vi "SubPanel_PowerConfiguration_Rev11_v4.vi"(3 "error in":errorcluster, 4 "VISAPowerInfoInputArray":T2[](array[typedef]), 5 "DCPowerInformationClusterArray_Input":T1[](array[typedef])) -> (0 "error out":errorcluster, 1 "VISAPowerInfoOutputArray":T2[](array[typedef]), 2 "DCPowerInformationClusterArray_Output":T1[](array[typedef]))   [LabVIEW 2019]
uses:
  Controls/PlotColorArray.ctl
  Controls/VISA_power_Control.ctl
  Controls/DCPowerBlock_byInstrument_Control.ctl
panel:
  out "DCPowerInformationClusterArray":T1[](array[typedef])
  out "VISAPowerInformationClusterArray":T2[](array[typedef])
  out "Current Measurement (A)":dbl[][](array[numeric])
  out "Voltage Measurement (V)":dbl[][](array[numeric])
  out "Voltage Waveform Array":waveform(dbl)[](graph)
  out "Current Waveform Array":waveform(dbl)[](graph)
  out "Supplies Updated?":bool
  in  "Update Changes":bool
  out "VISAPowerInformationClusterOutput":T3(array[cluster])
  in  "Exit SubVI":bool
  in  "Instrument Cards (Must Reconfigure if you add new cards or change the names in NI Max)":T4(tab)
  in  "VISA resource name":refnum<visa-resource-name>
  in  "Apply Power Settings":bool
  out "POWER STATUS":bool
  in  "POWER ON":bool
  in  "Voltage Channel 1":dbl
  in  "Voltage Channel 2":dbl
  in  "Voltage Channel 3":dbl
  in  "Current Limit Channel 1":dbl
  in  "Current Limit Channel 2":dbl
  in  "Current Limit Channel 3":dbl
  out "Parameter Configuration Echo":string[][](array[string])
  out "Configuration Echo":string
  in  "Which Channels to Parallelize":u16(ring) items=["I1+I2", "ALL", "I2+I3"]
  in  "Combination Scheme":u16(ring) items=["OFF", "SERIES", "PARALLEL"]
  in  "Current Reset Value 23":dbl
  in  "Current Reset Value 22":dbl
  in  "Current Reset Value 21":dbl
  in  "Current Reset Value 20":dbl
  in  "Current Reset Value 19":dbl
  in  "Current Reset Value 18":dbl
  in  "Current Reset Value 17":dbl
  in  "Current Reset Value 16":dbl
  in  "Current Reset Value 15":dbl
  in  "Current Reset Value 14":dbl
  in  "Current Reset Value 13":dbl
  in  "Current Reset Value 12":dbl
  in  "Current Reset Value 11":dbl
  in  "Current Reset Value 10":dbl
  in  "Current Reset Value 9":dbl
  in  "Current Reset Value 8":dbl
  in  "Current Reset Value 7":dbl
  in  "Current Reset Value 6":dbl
  in  "Current Reset Value 5":dbl
  in  "Current Reset Value 4":dbl
  in  "Current Reset Value 3":dbl
  in  "Current Reset Value 2":dbl
  in  "Current Reset Value 1":dbl
  in  "voltage level channel 26":dbl caption="voltage level channel 0" format="%.6p"
  in  "voltage level channel 1":dbl format="%.6p"
  in  "voltage level channel 2":dbl format="%.6p"
  in  "voltage level channel 3":dbl format="%.6p"
  in  "voltage level channel 4":dbl format="%.6p"
  in  "voltage level channel 5":dbl format="%.6p"
  in  "voltage level channel 6":dbl format="%.6p"
  in  "voltage level channel 7":dbl format="%.6p"
  in  "voltage level channel 8":dbl format="%.6p"
  in  "voltage level channel 9":dbl format="%.6p"
  in  "voltage level channel 10":dbl format="%.6p"
  in  "voltage level channel 11":dbl format="%.6p"
  in  "voltage level channel 12":dbl format="%.6p"
  in  "voltage level channel 13":dbl format="%.6p"
  in  "voltage level channel 14":dbl format="%.6p"
  in  "voltage level channel 15":dbl format="%.6p"
  in  "voltage level channel 16":dbl format="%.6p"
  in  "voltage level channel 17":dbl format="%.6p"
  in  "voltage level channel 18":dbl format="%.6p"
  in  "voltage level channel 19":dbl format="%.6p"
  in  "voltage level channel 20":dbl format="%.6p"
  in  "voltage level channel 21":dbl format="%.6p"
  in  "voltage level channel 22":dbl format="%.6p"
  in  "voltage level channel 23":dbl format="%.6p"
  in  "Activate Channel 0":bool
  in  "Activate Channel 1":bool
  in  "Activate Channel 2":bool
  in  "Activate Channel 3":bool
  in  "Activate Channel 4":bool
  in  "Activate Channel 5":bool
  in  "Activate Channel 6":bool
  in  "Activate Channel 7":bool
  in  "Activate Channel 8":bool
  in  "Activate Channel 9":bool
  in  "Active Channel 10":bool
  in  "Activate Channel 11":bool
  in  "Activate Channel 12":bool
  in  "Activate Channel 13":bool
  in  "Activate Channel 14":bool
  in  "Activate Channel 15":bool
  in  "Activate Channel 16":bool
  in  "Activate Channel 17":bool
  in  "Activate Channel 18":bool
  in  "Activate Channel 19":bool
  in  "Activatate Channel 20":bool
  in  "Activate Channel 21":bool
  in  "Activate Channel 22":bool
  in  "Activate Channel 23":bool
  in  "Channel Name 0":string="NULL0"
  in  "Channel Name 1":string="NULL1"
  in  "Channel Name 2":string="NULL2"
  in  "Channel Name 3":string="NULL3"
  in  "Channel Name 4":string="NULL4"
  in  "Channel Name 5":string="NULL5"
  in  "Channel Name 6":string="NULL6"
  in  "Channel Name 7":string="NULL7"
  in  "Channel Name 8":string="NULL8"
  in  "Channel Name 9":string="NULL9"
  in  "Channel Name 10":string="NULL10"
  in  "Channel Name 11":string="NULL11"
  in  "Channel Name 12":string="NULL12"
  in  "Channel Name 13":string="NULL13"
  in  "Channel Name 14":string="NULL14"
  in  "Channel Name 15":string="NULL15"
  in  "Channel Name 16":string="NULL16"
  in  "Channel Name 17":string="NULL17"
  in  "Channel Name 18":string="NULL18"
  in  "Channel Name 19":string="NULL19"
  in  "Channel Name 20":string="NULL20"
  in  "Channel Name 21":string="NULL21"
  in  "Channel Name 22":string="NULL22"
  in  "Channel Name 23":string="NULL23"
  in  "Apply Power Settings":bool
  in  "Aperture Time (s)":dbl=0.0001
  in  "Measure Record Length":i32=1000000
  in  "current limit (A) 2":dbl=0.05
  out "All Channel Numbers Array 2":string[](array[string])=["0", "1", "2", "3", "4", "5", "6", "7", "8", "9", "10", "11", "12", "13", "14", "15", "16", "17", "18", "19", "20", "21", "22", "23"]
  out "Active Channels Indicator 2":bool[](array[boolean])
  out "Voltage Array":dbl[](array[numeric])
  out "Active Channel Numbers Array 2":string[](array[string])
  out "Active Channel Voltage Array":dbl[](array[numeric])
  out "Active Channel Names Array":string[](array[string])
  in  "Current Reset Value 0":dbl
  in  "voltage level channel 0":dbl=1.0 format="%.6p"
  in  "Activate Channel 0":bool
  in  "Queue Power Settings":bool
  in  "Channel Name 0":string="NULL_0_slot16"
  out "Active Channel Voltage Array 3":dbl[](array[numeric])
  out "Active Channels Indicator 3":bool[](array[boolean])
  out "Voltage Array":dbl[](array[numeric])=[1.0]
  out "Active Channel Names Array":string[](array[string])
  out "Active Channel Numbers Array 3":string[](array[string])
  out "All Channel Numbers Array 3":string[](array[string])=["0"]
  in  "current limit (A) 3":dbl=3.0
  in  "Measure Record Length":i32=1000000
  in  "Aperture Time (s)":dbl=0.001
  in  "Current Reset Value 0":dbl
  in  "Queue Power Settings":bool
  in  "Aperture Time (s)":dbl=0.001
  in  "Measure Record Length":i32=1000000
  in  "current limit (A) 4":dbl=3.0
  in  "Activate Channel 0":bool
  in  "voltage level channel 0":dbl=2.0 format="%.6p"
  in  "Channel Name 0":string="NULL_0_slot_16"
  out "Active Channel Names Array":string[](array[string])
  out "Active Channel Voltage Array 4":dbl[](array[numeric])
  out "Active Channel Numbers Array 4":string[](array[string])
  out "Voltage Array":dbl[](array[numeric])=[2.0]
  out "Active Channels Indicator 4":bool[](array[boolean])
  out "All Channel Numbers Array 4":string[](array[string])=["0"]
  in  "Current Reset Value 0":dbl
  in  "Current Reset Value 0":dbl
  out "Active Channel Names Array":string[](array[string])
  out "Active Channel Voltage Array":dbl[](array[numeric])
  out "Active Channel Numbers Array":string[](array[string])
  out "Voltage Array":dbl[](array[numeric])=[3.0]
  out "All Channel Numbers Array":string[](array[string])=["0"]
  out "Active Channels Indicator":bool[](array[boolean])
  in  "voltage level channel 0":dbl=3.0 format="%.6p"
  in  "Activate Channel 0":bool
  in  "Channel Name 0":string="NULL_0_slot16"
  in  "Queue Power Settings":bool
  in  "Aperture Time (s)":dbl=0.001
  in  "Measure Record Length":i32=1000000
  in  "current limit (A)":dbl=3.0
  out "DCPowerInformationClusterOutput":T5(array[cluster])
  in  "ColorPalette":T6=[16711686, 65351, 8978420, 14474240, 16139007, 16752640, 8958719, 16758973, 16777215, 46792, 11992992, 12961221, 16763690, 12600063, 16711835, 2953983, 40796, 13111296, 13352613, 9221011, 12964076, 12819897, 65442, 16776704, 14540253, 16740729, 10658047, 10813344, 16753521, 13413843, 8691115, 10339240, 14401205, 16746704, 7467519, 16775978, 13872558, 11387603, 13354405, 10420227, 13107364, 4060, 35208, 11817216, 7566080, 40796, 7539456, 2837073, 6372186, 7499083, 10648702, 16757152]
  # "Background Information (Important)\nThis subvi has tabs that allow you to configure different power instruments. There are two options: VISA instruments or DC Power instruments. DC Power instruments are inside of the tester, visa instruments are external. If DCPower instruments are switched out, they will need to be reconfigured within the backend of this code (instructions pending). You are able to identify which channels you want to active, their individual voltage levels and the desired \"name\" of the channel (i.e. if you want channel 0 to be known at the \"ADMV1013_3p3V\" or \"GoodEnough\", you write it here). For the entire instrument, you can determine its capture rate (aperture time) or the current limit. I advise you do NOT alter the \"Measure Record Length\" as this is only if there are issues with the program. Shouldn't ever exceed this value. You apply the settings and they will be echoed back in each tab along with the array above. Multiple instruments can be configured and will show up as separate array elements\n\n\nInstructions (More Important):\n\nSelect instrument of interest (VISA KEITHLEY 2230G-30-6, PXIe-4163, and PXIe-4139 are the ones currently available). \n\n\nFOR DCPOWER INSTRUMENTS (PXI or PXIe)\n\nPress \"Active Channel #\" to select which channels you want to have power applied \n\nType in voltage level in \"Voltage level channel #\"\n\nType in desired channel name in \"Channel Name #\"\n\nType the measurement speed (suggest .0001) in aperture time\n\nType the current limit in \"current limit\"\n\nPress \"Apply Power Settings\" and review the echoed outputs within the tab and in the instrument array above the tabs.\n\nRepeat this process for other instruments\n\n\n\nFOR VISA INSTRUMENTS (NOT PXI or PXIe), note that it is case by case for instruments\n\nSelect resource name (you must know which one it is)\n\nPower on device if using it\n\nApply voltage settings \n\nApply current limits for each channel\n\nSelect which channels you will parallelize if at all\n\nSelect which combination scheme you will apply: OFF (individual channels), SERIES (Channel 1 and 2 in series), PARALLEL (I1 + I2, ALL, I2 + I3)\n\nFOR COMBINATIONS: for a combination scheme you choose, you only apply changes to the first channel of each. example: if you make the system series configuration, you only type you voltage information (i.e. 60V) into channel 1 and the current limit information into channel 1 but channel 3 is still independent of these\n\n\nPress \"Apply Powe Settings\" when complete\n\nReview the echoed values along with the instrument array above"
  # "All Voltage Level Channels are in Volts"
  # "Don't press enter when typing in strings. Just click out of it"
  # "Don't press enter when typing in strings. Just click out of it"
  # "Don't press enter when typing in strings. Just click out of it"
  # "Don't press enter when typing in strings. Just click out of it"
  # "Don't press enter when typing in strings. Just click out of it"
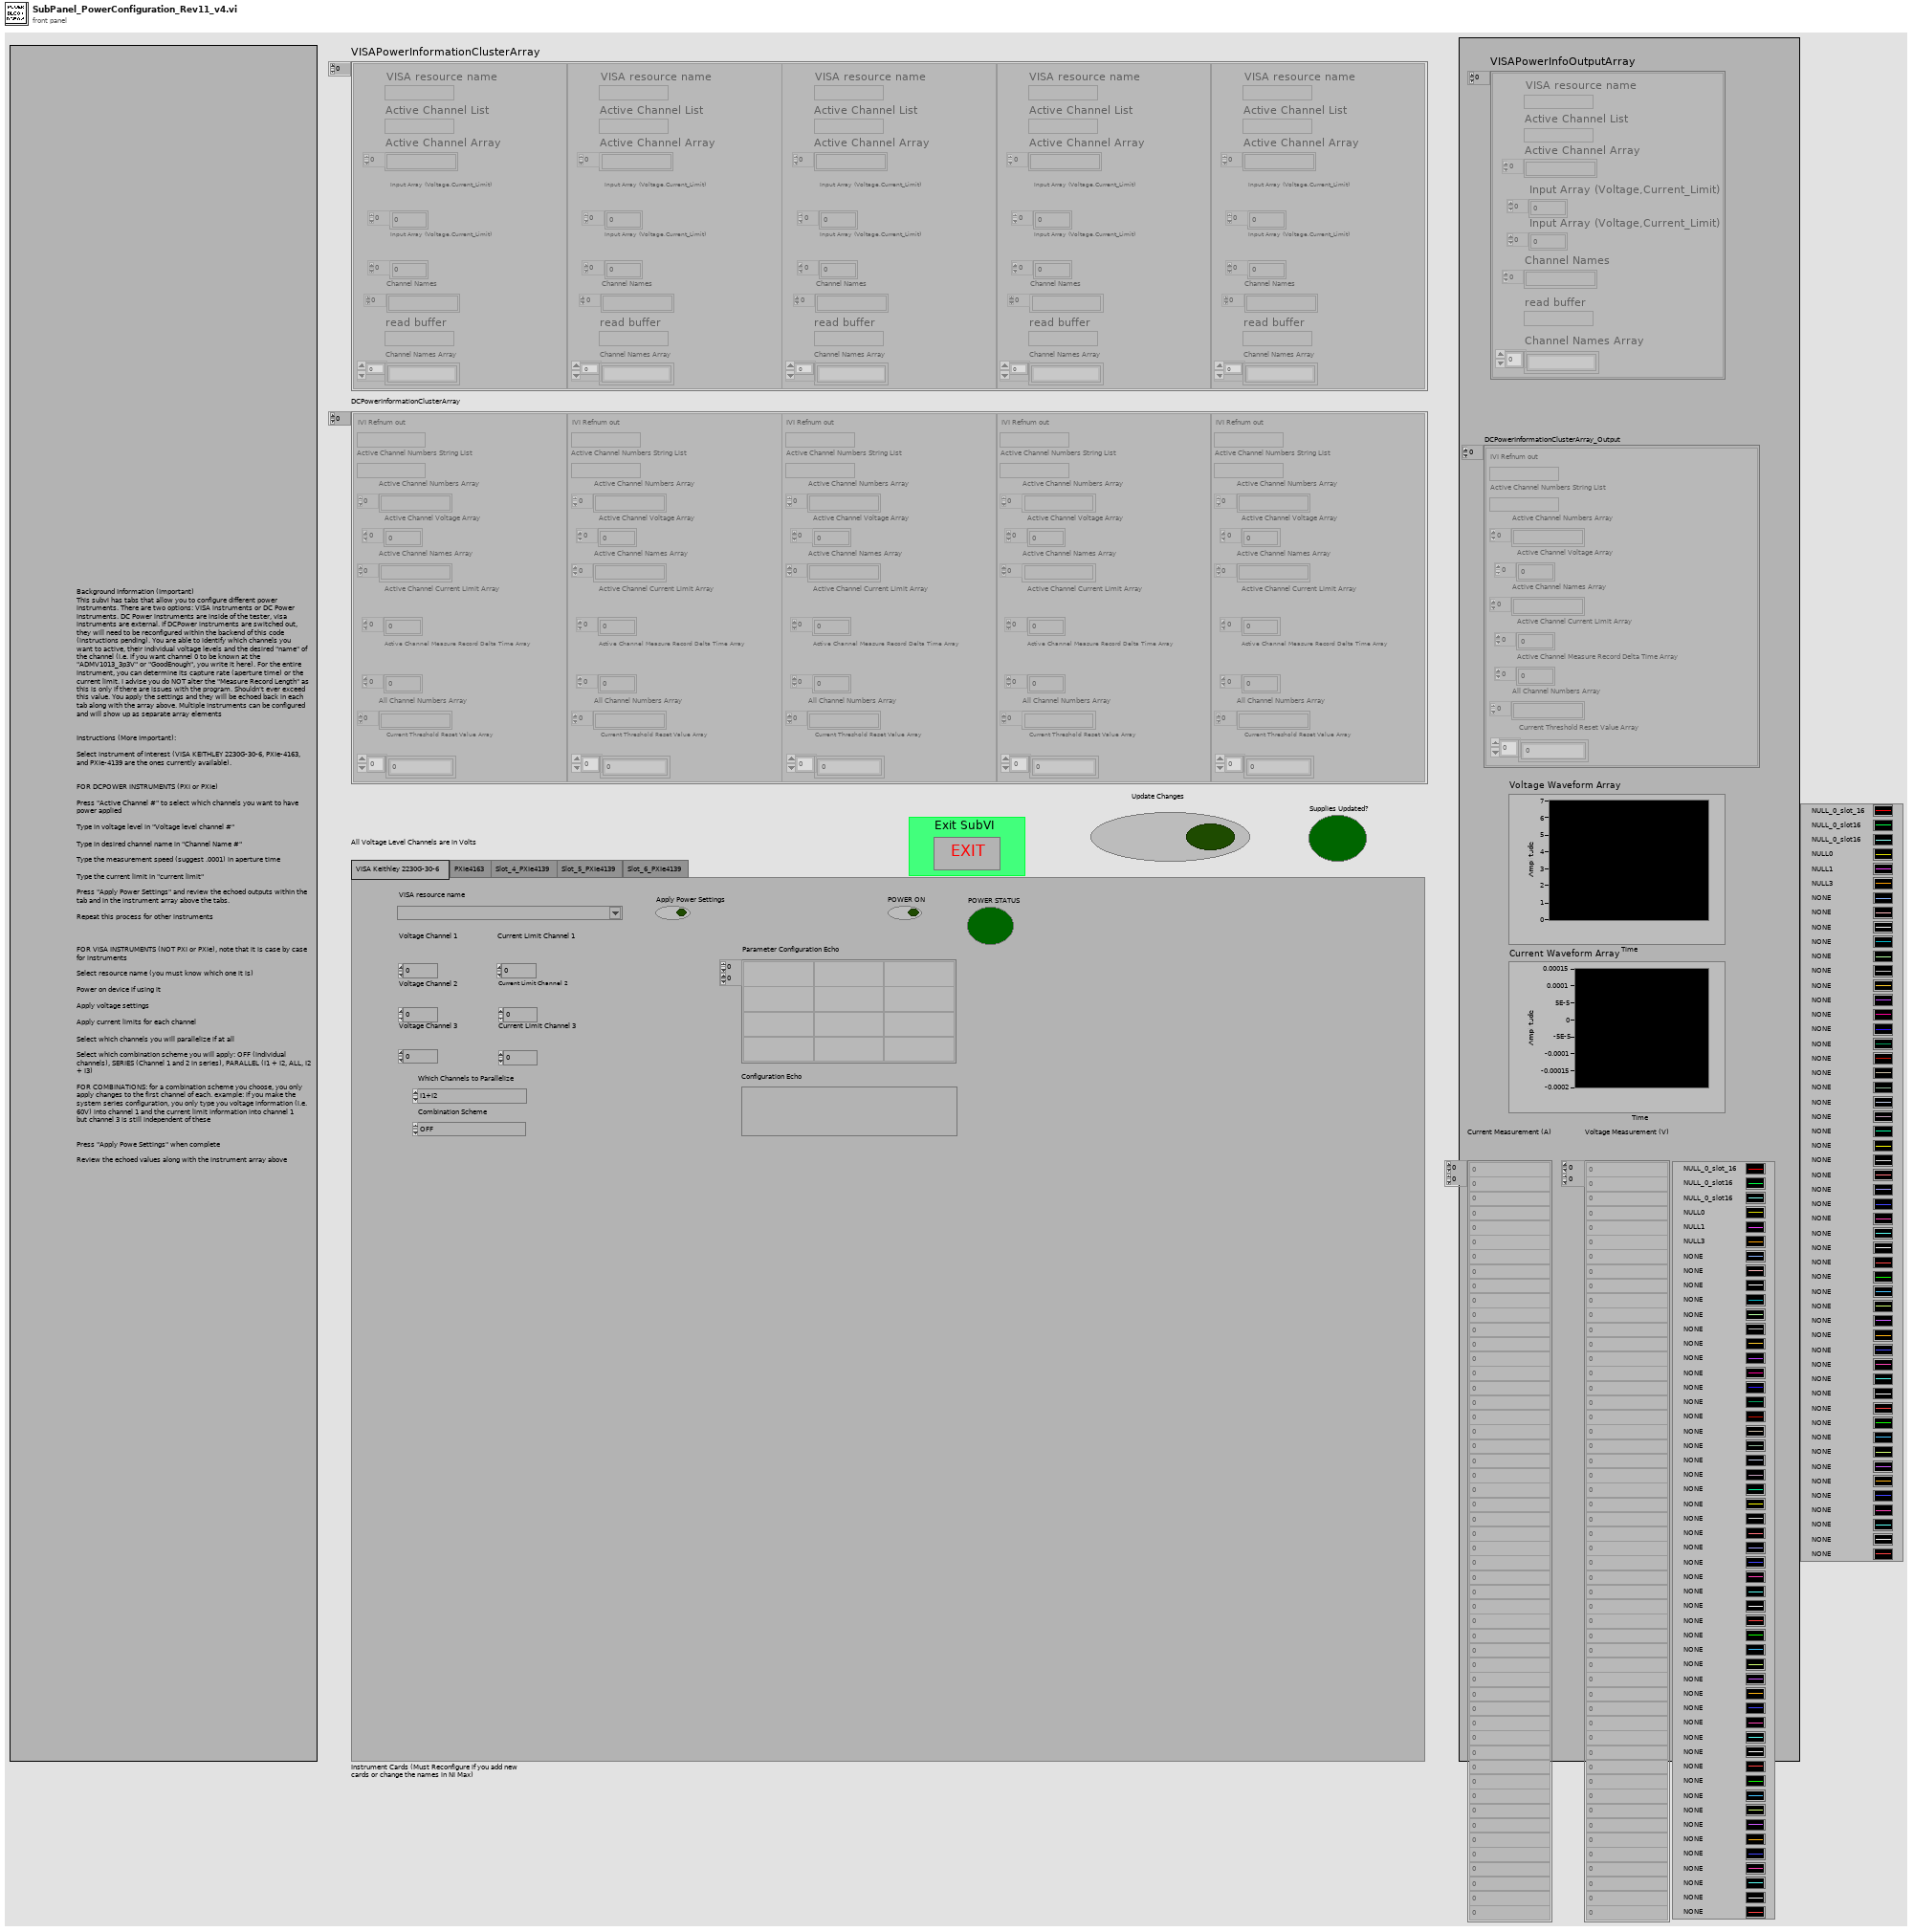
[diagram p1: front panel]
types:
  T1 = typedef "DCPowerBlock_byInstrument_Control.ctl" = cluster{"IVI Refnum out":refnum<k15>, "Active Channel Numbers String List":string, "Active Channel Numbers Array":string[], "Active Channel Voltage Array":dbl[], "Active Channel Names Array":string[], "Active Channel Current Limit Array":dbl[], "Active Channel Measure Record Delta Time Array":dbl[], "All Channel Numbers Array":string[], "Current Threshold Reset Value Array":dbl[]}
  T2 = typedef "VISA_power_Control.ctl" = cluster{"VISA resource name":refnum<visa-resource-name>, "Active Channel List":string, "Active Channel Array":string[], "Input Array (Voltage,Current_Limit)":dbl[], "Input Array (Voltage,Current_Limit)":dbl[], "Channel Names":string[], "read buffer":string, "Channel Names Array":string[]}
  T3 = cluster{"VISA resource name":refnum<visa-resource-name>, "String List":string, string[], "Input Array (Voltage,Current_Limit)":dbl[], "Input Array (Voltage,Current_Limit)":dbl[], "Channel Names":string[]}[]
  T4 = enum32{"VISA Keithley 2230G-30-6", "PXIe4163", "Slot_4_PXIe4139", "Slot_5_PXIe4139", "Slot_6_PXIe4139"}
  T5 = cluster{"instrument handle out":refnum<k15>, string, string[], dbl[], string[]}[]
  T6 = typedef "PlotColorArray.ctl" = u32[]
  T7 = cluster{"IVI Refnum out":refnum<k15>, "Active Channel Numbers String List":string, "Active Channel Numbers Array":string[], "Active Channel Voltage Array":dbl[], "Active Channel Names Array":string[], "Active Channel Current Limit Array":dbl[], "Active Channel Measure Record Delta Time Array":dbl[], "All Channel Numbers Array":string[]}[]
  T8 = cluster{"instrument handle out":refnum<k15>, string, string[], dbl[], string[], "Current Limit Output Array":dbl[], dbl[]}[]
  T9 = cluster{"IVI Refnum out":refnum<k15>, "Active Channel Numbers String List":string, "Active Channel Numbers Array":string[], "Active Channel Voltage Array":dbl[], "Active Channel Names Array":string[], "Active Channel Current Limit Array":dbl[], "Active Channel Measure Record Delta Time Array":dbl[], "All Channel Numbers Array":string[]}
  T10 = cluster{"VISA resource name":refnum<visa-resource-name>, "String List":string, string[], "Input Array (Voltage,Current_Limit)":dbl[], "Input Array (Voltage,Current_Limit)":dbl[], "Channel Names":string[], "read buffer":string}[]
  T11 = cluster{"IVI Refnum out":refnum<k15>, "Active Channel Numbers String List":string, "Active Channel Numbers Array":string[], "Active Channel Voltage Array":dbl[], "Active Channel Names Array":string[], "Active Channel Current Limit Array":dbl[], "Active Channel Measure Record Delta Time Array":dbl[], "aperture time string":string[], dbl[]}
  T12 = cluster{"IVI Refnum out":refnum<k15>, "Active Channel Numbers String List":string, "Active Channel Numbers Array":string[], "Active Channel Voltage Array":dbl[], "Active Channel Names Array":string[], "Active Channel Current Limit Array":dbl[], "Active Channel Measure Record Delta Time Array":dbl[], "All Channel Numbers Array":string[], dbl[]}
  T13 = cluster{"IVI Refnum out":refnum<k15>, string, "voltage level channel 23":dbl, "Channel Name 23":string, "Current Limit":dbl, "Measure Record dt":dbl, string, "Current Threshold Reset Value Array":dbl}[]
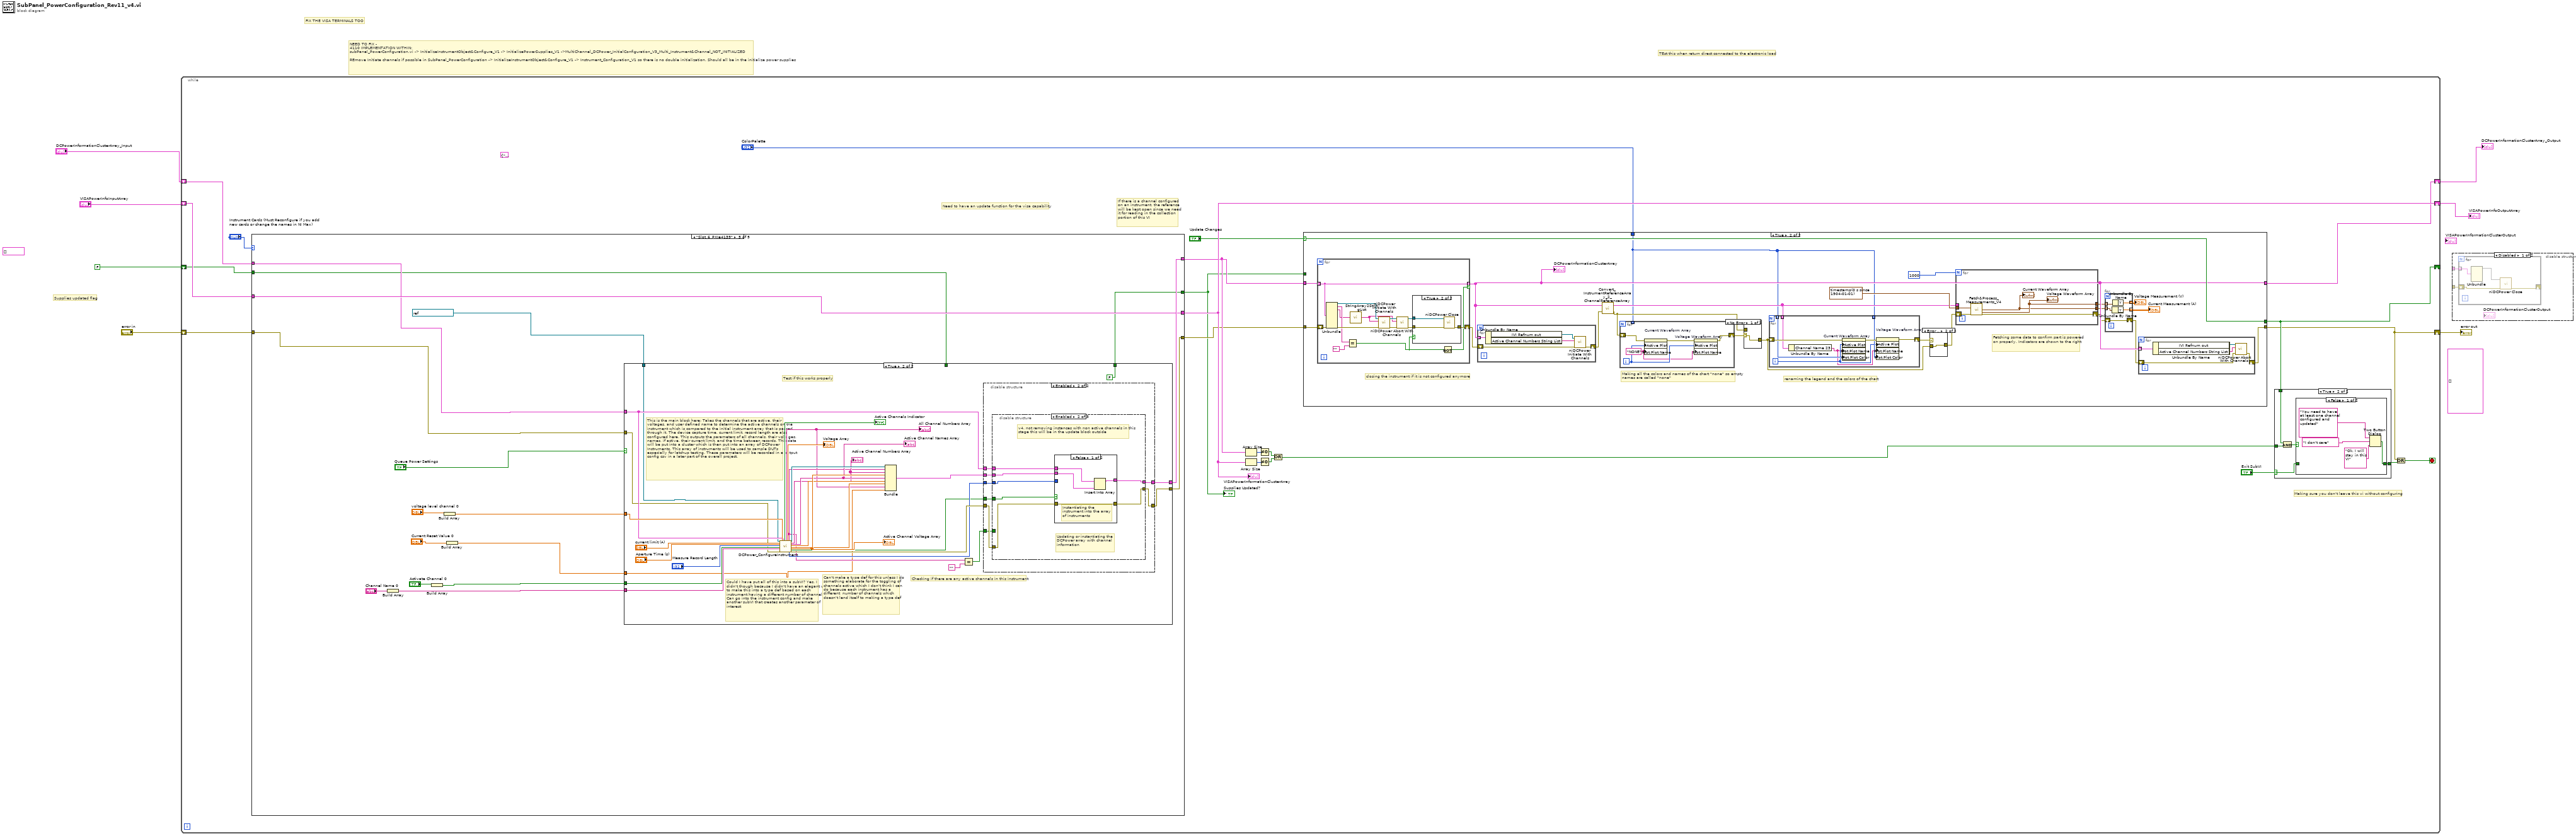
[diagram p0: block diagram]
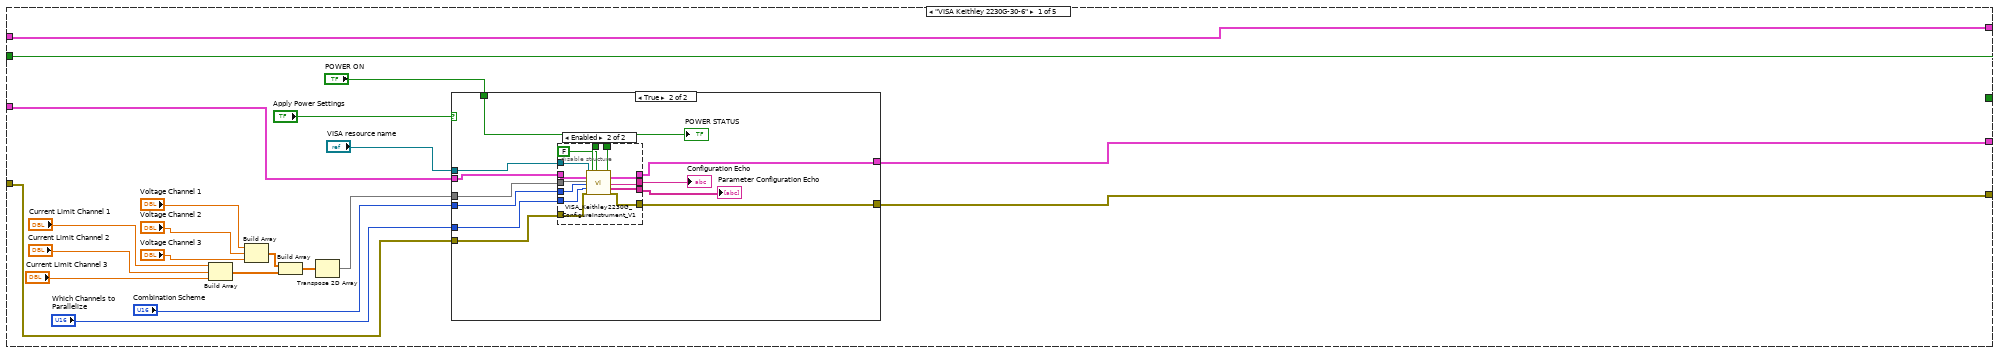
[diagram p9: hidden frame]
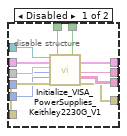
[diagram p11: hidden frame]
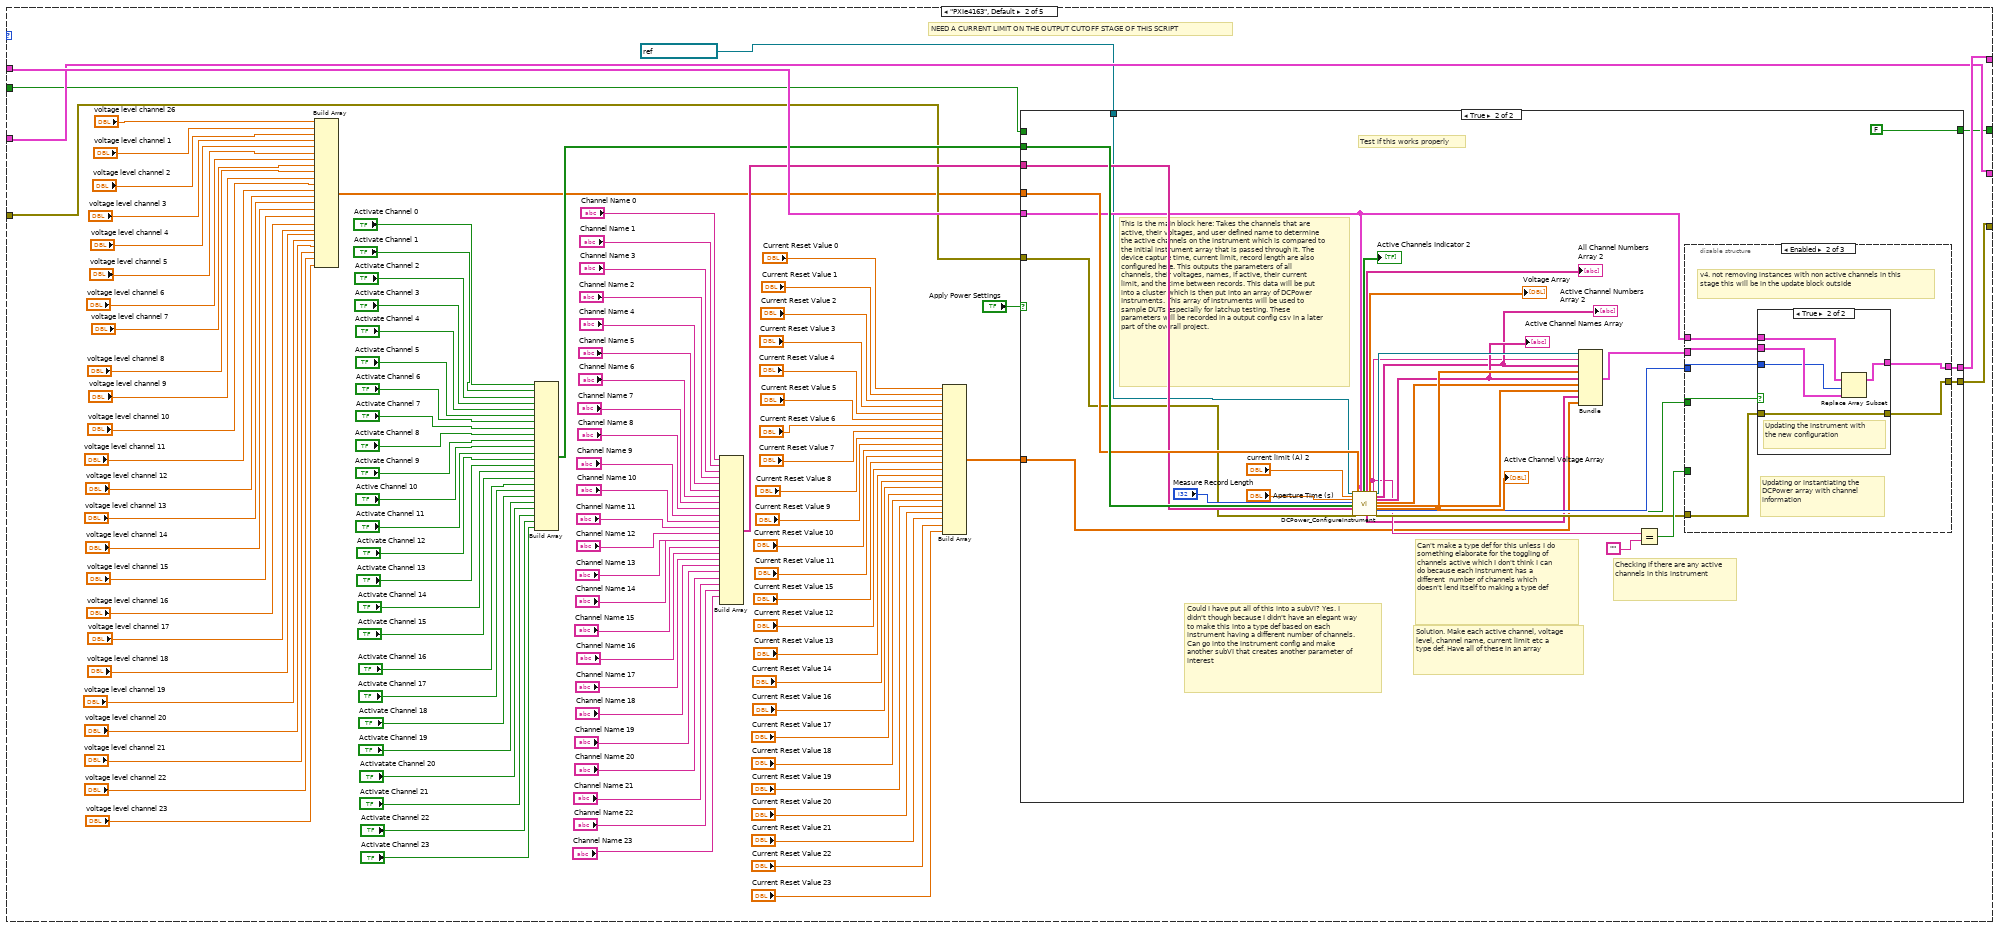
[diagram p12: hidden frame]
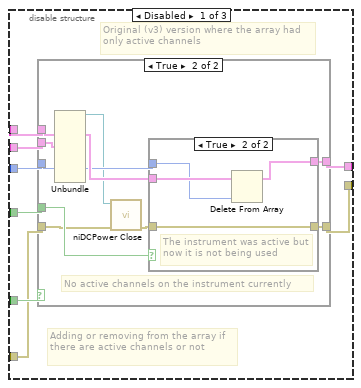
[diagram p14: hidden frame]
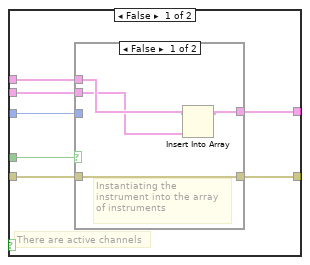
[diagram p15: hidden frame]
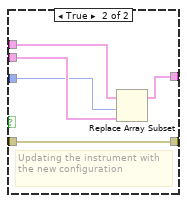
[diagram p16: hidden frame]
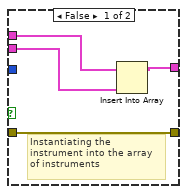
[diagram p18: hidden frame]
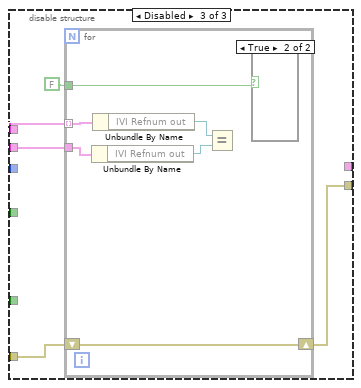
[diagram p19: hidden frame]
diagram:
  (unwired) T7 []
  (unwired) T8 [] ("DCPowerInformationClusterArray_Input")
  # "Supplies updated flag"
  # "TEst this when return direct connected to the electronic load"
  # "FIX THE VISA TERMINALS TOO"
  # "NEED TO FIX - \n4110 IMPLEMENTATION WITHIN:\nsubPanel_PowerConfiguration.vi -> InitializeInstrumentObject&Configure_V1 -> InitializePowerSupplies_V1 ->MultiChannel_DCPower_InitialConfiguration_V3_Multi_Instrument&Channel_NOT_INITIALIZED\n\nREmove Initiate channels if possible in SubPanel_PowerConfiguration -> InitializeInstrumentObject&Configure_V1 -> Instrument_Configuration_V1 so there is no double initialization. Should all be in the initialize power supplies"
  n1 = while {
    shift-right: [w22] -> w5
    shift-left: "DCPowerInformationClusterArray_Input" -> [w24]
    shift-right: [w21] -> w6
    shift-left: "error in" -> [w23]
    shift-right: [w28] -> w2
    shift-left: "VISAPowerInfoInputArray" -> [w29]
    shift-right: [w25] -> _
    shift-left: FALSE -> [w26]
    stop <- w27 stop-if-true
    (unwired) T9 {"IVI Refnum out"="", "Active Channel Numbers String List"="", "Active Channel Numbers Array"=[], "Active Channel Voltage Array"=[], "Active Channel Names Array"=[], "Active Channel Current Limit Array"=[], "Active Channel Measure Record Delta Time Array"=[], "All Channel Numbers Array"=[]} ("output cluster")
    # "Making sure you don't leave this vi without configuring"
    # "Need to have an update function for the visa capability"
    # "If there is a channel configured on an instrument, the reference will be kept open since we need it for reading in the collection portion of this VI"
    n2 = case shown="\"Slot_6_PXIe4139\"" "Instrument Cards (Must Reconfigure if you add new cards or change the names in NI Max)" {
      tunnel: w24 -> [w138 w217 w393 w555 w717]
      tunnel: w23 -> [w126 w214 w401 w563 w725]
      tunnel: [w123 w213 w395 w557 w719] -> w9
      tunnel: [w138 w212 w396 w558 w720] -> w11
      tunnel: w29 -> [w139 w211 w394 w556 w718]
      tunnel: [w122 w211 w394 w556 w718] -> w28
      tunnel: [w121 w209 w392 w553 w716] -> w8
      tunnel: w26 -> [w121 w208 w391 w554 w715]
      frame "VISA Keithley 2230G-30-6" {
        n3 = Build Array("Current Limit Channel 1", "Current Limit Channel 2", "Current Limit Channel 3") -> (w136:dbl[])
        n4 = Build Array("Voltage Channel 1", "Voltage Channel 2", "Voltage Channel 3") -> (w135:dbl[])
        n5 = Build Array(w135, w136) -> (w137:dbl[][])
        n6 = Transpose 2D Array(2D array=w137) -> (transposed array=w127:dbl[][])
        n7 = case shown="True" "Apply Power Settings" {
          tunnel: "VISA resource name" -> [_ w155]
          tunnel: w139 -> [w142 w154]
          tunnel: "POWER ON" -> [_ w153]
          tunnel: w127 -> [_ w152]
          tunnel: w126 -> [w143 w151]
          tunnel: "Which Channels to Parallelize" -> [_ w150]
          tunnel: "Combination Scheme" -> [_ w149]
          tunnel: [w142 w145] -> w122
          tunnel: [w143 w144] -> w123
          frame False {
          }
          frame True {
            n8 = disable-structure shown="Enabled" {
              disable-tunnel: w155 -> [w167 w178]
              disable-tunnel: w154 -> [w166 w177]
              disable-tunnel: w153 -> [w165 w179]
              disable-tunnel: w152 -> [w164 w176]
              disable-tunnel: w151 -> [w163 w173]
              disable-tunnel: w150 -> [w162 w174]
              disable-tunnel: w149 -> [w161 w175]
              disable-tunnel: [w160 w180] -> w148
              disable-tunnel: [w159 w171] -> w147
              disable-tunnel: [w158 w170] -> w146
              disable-tunnel: [w157 w172] -> w145
              disable-tunnel: [w156 w169] -> w144
              frame Disabled {
                n9 = call "Initialize_VISA_PowerSupplies_Keithley2230G_V1.vi"("VISA resource name"=w167, "VISAPowerInfoInputArray"=w166, "Input Array (Voltage,Current_Limit)"=w164, "Combination Scheme"=w161, "Which Channels to Parallelize"=w162, "error in"=w163, "POWER STATUS IN"=w165) -> ("POWER STATUS OUT"=w160:bool, "VISAPowerInfoOutputArray"=w157:T10, "Configuration Echo"=w159:string, "Parameter Configuration Echo"=w158:string[][], "error out"=w156:errorcluster)  [unwired: 8 in]
              }
              frame Enabled {
                n10 = call "VISA_Keithley2230G_ConfigureInstrument_V1.vi"("VISA resource name"=w178, "VISAPowerInfoInputArray"=w177, "Input Array (Voltage,Current_Limit)"=w176, "Combination Scheme"=w175, "Which Channels to Parallelize"=w174, "error in"=w173, "POWER STATUS IN"=w179, "json configured?"=FALSE) -> ("POWER STATUS OUT"=w180:bool, "VISAPowerInfoOutputArray"=w172:T2[], "Configuration Echo"=w171:string, "Parameter Configuration Echo"=w170:string[][], "error out"=w169:errorcluster)  [unwired: 7 in]
              }
            }
            "POWER STATUS" <- w148
            "Configuration Echo" <- w147
            "Parameter Configuration Echo" <- w146
          }
        }
      }
      frame "PXIe4163", Default {
        # "NEED A CURRENT LIMIT ON THE OUTPUT CUTOFF STAGE OF THIS SCRIPT"
        n11 = Build Array("voltage level channel 26", "voltage level channel 1", "voltage level channel 2", "voltage level channel 3", "voltage level channel 4", "voltage level channel 5", "voltage level channel 6", "voltage level channel 7", "voltage level channel 8", "voltage level channel 9", "voltage level channel 10", "voltage level channel 11", "voltage level channel 12", "voltage level channel 13", "voltage level channel 14", "voltage level channel 15", "voltage level channel 16", "voltage level channel 17", "voltage level channel 18", "voltage level channel 19", "voltage level channel 20", "voltage level channel 21", "voltage level channel 22", "voltage level channel 23") -> (w210:dbl[])
        n12 = Build Array("Activate Channel 0", "Activate Channel 1", "Activate Channel 2", "Activate Channel 3", "Activate Channel 4", "Activate Channel 5", "Activate Channel 6", "Activate Channel 7", "Activate Channel 8", "Activate Channel 9", "Active Channel 10", "Activate Channel 11", "Activate Channel 12", "Activate Channel 13", "Activate Channel 14", "Activate Channel 15", "Activate Channel 16", "Activate Channel 17", "Activate Channel 18", "Activate Channel 19", "Activatate Channel 20", "Activate Channel 21", "Activate Channel 22", "Activate Channel 23") -> (w216:bool[])
        n13 = Build Array("Channel Name 0", "Channel Name 1", "Channel Name 3", "Channel Name 2", "Channel Name 4", "Channel Name 5", "Channel Name 6", "Channel Name 7", "Channel Name 8", "Channel Name 9", "Channel Name 10", "Channel Name 11", "Channel Name 12", "Channel Name 13", "Channel Name 14", "Channel Name 15", "Channel Name 16", "Channel Name 17", "Channel Name 18", "Channel Name 19", "Channel Name 20", "Channel Name 21", "Channel Name 22", "Channel Name 23") -> (w215:string[])
        n14 = Build Array("Current Reset Value 0", "Current Reset Value 1", "Current Reset Value 2", "Current Reset Value 3", "Current Reset Value 4", "Current Reset Value 5", "Current Reset Value 6", "Current Reset Value 7", "Current Reset Value 8", "Current Reset Value 9", "Current Reset Value 10", "Current Reset Value 11", "Current Reset Value 15", "Current Reset Value 12", "Current Reset Value 13", "Current Reset Value 14", "Current Reset Value 16", "Current Reset Value 17", "Current Reset Value 18", "Current Reset Value 19", "Current Reset Value 20", "Current Reset Value 21", "Current Reset Value 22", "Current Reset Value 23") -> (w181:dbl[])
        n15 = case shown="True" "Apply Power Settings" {
          tunnel: w217 -> [w292 w307]
          tunnel: refnum<k15> "PXIe4163" ("resource name") -> [_ w295]
          tunnel: w216 -> [_ w322]
          tunnel: w215 -> [_ w320]
          tunnel: w214 -> [w291 w296]
          tunnel: [w291 w305] -> w213
          tunnel: [w292 w304] -> w212
          tunnel: w210 -> [_ w321]
          tunnel: [w290 FALSE] -> w209
          tunnel: w208 -> [w290 _]
          tunnel: w181 -> [_ w293]
          frame False {
          }
          frame True {
            # "Solution. Make each active channel, voltage level, channel name, current limit etc a type def. Have all of these in an array"
            # "This is the main block here: Takes the channels that are active, their voltages, and user defined name to determine the active channels on the instrument which is compared to the initial instrument array that is passed through it. The device capture time, current limit, record length are also configured here. This outputs the parameters of all channels, their voltages, names, if active, their current limit, and the time between records. This data will be put into a cluster which is then put into an array of DCPower Instruments. This array of instruments will be used to sample DUTs especially for latchup testing. These parameters will be recorded in a output config csv in a later part of the overall project."
            # "Checking if there are any active channels in this instrument"
            # "Could I have put all of this into a subVI? Yes. I didn't though because I didn't have an elegant way to make this into a type def based on each instrument having a different number of channels. Can go into the instrument config and make another subVI that creates another parameter of interest"
            # "Can't make a type def for this unless I do something elaborate for the toggling of channels active which I don't think I can do because each instrument has a different  number of channels which doesn't lend itself to making a type def"
            # "Test if this works properly"
            n16 = call "DCPower_ConfigureInstrument.vi"("IVI Refnum in"=w295, "current limit"="current limit (A) 2", "Aperture Time"="Aperture Time (s)", "Measure Record Length"="Measure Record Length", "Active Channels Input"=w322, "Channel Name Array"=w320, "error in (no error)"=w296, "Voltage Array Input"=w321, "DCPowerInformationClusterArray_Input"=w307) -> ("Active Channels Indicator"=→"Active Channels Indicator 2":bool[], "All Channel Numbers Array"=→"All Channel Numbers Array 2":string[], "aperture time string"=w294:string[], "Total Voltage Indicator Array"=→"Voltage Array":dbl[], "Active Channel Numbers String List"=w299:string, "IVI Ref index"=w303:i32, "IVI Refnum out"=w315:refnum<k15>, "Active Channel Numbers Array"=w301:string[], "Active Channel Names Array"=w313:string[], "Active Channel Current Limit Array"=w312:dbl[], "Active Channel Measure Record Delta Time Array"=w311:dbl[], "Active Channel Voltage Array"=w314:dbl[], "IVI Ref Present?"=w302:bool, "error out"=w306:errorcluster)  [unwired: 4 in, 1 out]
            "Active Channel Numbers Array 2" <- w301
            "Active Channel Names Array" <- w313
            "Active Channel Voltage Array" <- w314
            n17 = Bundle("IVI Refnum out"=w315, "Active Channel Numbers String List"=w299, "Active Channel Numbers Array"=w301, "Active Channel Voltage Array"=w314, "Active Channel Names Array"=w313, "Active Channel Current Limit Array"=w312, "Active Channel Measure Record Delta Time Array"=w311, "aperture time string"=w294, w293) -> (w308:T11)  [unwired: 1 in]
            n18 = Equal?(x=w299, y="") -> (x = y?=w309:bool)
            n19 = disable-structure shown="Enabled" {
              disable-tunnel: w309 -> [w330 _ _]
              disable-tunnel: w308 -> [w329 w368 w379]
              disable-tunnel: w307 -> [w328 w367 w382]
              disable-tunnel: w306 -> [w327 w366 w380]
              disable-tunnel: [w326 w365 w381] -> w305
              disable-tunnel: [w325 w364 _] -> w304
              disable-tunnel: w303 -> [w324 w363 _]
              disable-tunnel: w302 -> [w323 w362 _]
              frame Disabled {
                # "Original (v3) version where the array had only active channels"
                # "Adding or removing from the array if there are active channels or not"
                n20 = case shown="True" w330 {
                  tunnel: w323 -> [w337 w354]
                  tunnel: [w336 w351] -> w325
                  tunnel: [w335 w352] -> w326
                  tunnel: w327 -> [w334 w349]
                  tunnel: w324 -> [w333 w353]
                  tunnel: w329 -> [w332 w347]
                  tunnel: w328 -> [w331 w355]
                  frame False {
                    # "There are active channels"
                    n21 = case shown="False" w337 {
                      tunnel: w331 -> [w340 w346]
                      tunnel: w332 -> [w339 w345]
                      tunnel: w333 -> [_ w344]
                      tunnel: w334 -> [w341 w343]
                      tunnel: [w341 w343] -> w335
                      tunnel: [w338 w342] -> w336
                      frame False {
                        # "Instantiating the instrument into the array of instruments"
                        n22 = Insert Into Array(array=w340, new element=w339) -> (w338:T1[])  [unwired: 1 in]
                      }
                      frame True {
                        # "Updating the instrument with the new configuration"
                        n23 = Replace Array Subset(array=w346, new element=w345, index=w344) -> (w342:T1[])
                      }
                    }
                  }
                  frame True {
                    # "No active channels on the instrument currently"
                    n24 = Unbundle(w347) -> ("IVI Refnum out"=w350:refnum<k15>)  [unwired: 8 out]
                    n25 = call <instrlib>:"niDCPower Close.vi"("error in (no error)"=w349, "instrument handle"=w350) -> ("error out"=w348:errorcluster)  [unwired: 9 in]
                    n26 = case shown="True" w354 {
                      tunnel: w355 -> [w357 w361]
                      tunnel: w353 -> [_ w360]
                      tunnel: [w356 w359] -> w352
                      tunnel: w348 -> [w356 w359]
                      tunnel: [w357 w358] -> w351
                      frame False {
                        # "The instrument wasn't active and it is still not being used"
                      }
                      frame True {
                        # "The instrument was active but now it is not being used"
                        n27 = Delete From Array(array=w361, index=w360) -> (array with subset deleted=w358:T1[])  [unwired: 1 in, 1 out]
                      }
                    }
                  }
                }
              }
              frame Enabled {
                # "v4. not removing instances with non active channels in this stage this will be in the update block outside"
                # "Updating or instantiating the DCPower array with channel information"
                n28 = case shown="True" w362 {
                  tunnel: w367 -> [w371 w377]
                  tunnel: w368 -> [w370 w376]
                  tunnel: w363 -> [_ w375]
                  tunnel: w366 -> [w372 w374]
                  tunnel: [w372 w374] -> w365
                  tunnel: [w369 w373] -> w364
                  frame False {
                    # "Instantiating the instrument into the array of instruments"
                    n29 = Insert Into Array(array=w371, new element=w370) -> (w369:T1[])  [unwired: 1 in]
                  }
                  frame True {
                    # "Updating the instrument with the new configuration"
                    n30 = Replace Array Subset(array=w377, new element=w376, index=w375) -> (w373:T1[])
                  }
                }
              }
              frame Disabled {
                n31 = for {
                  tunnel: w382 -> [w388] mode=indexing
                  shift-right: [w387] -> w381
                  shift-left: w380 -> [w387]
                  tunnel: w379 -> [w385]
                  tunnel: FALSE -> [w383]
                  n32 = Unbundle By Name(w385) -> ("IVI Refnum out"=w384:refnum<k15>)
                  n33 = Unbundle By Name(w388) -> ("IVI Refnum out"=w386:refnum<k15>)
                  n34 = Equal?(x=w386, y=w384) -> ()  [unwired: 1 out]
                  n35 = case shown="True" w383 {
                    frame False {
                    }
                    frame True {
                    }
                  }
                }
              }
            }
          }
        }
      }
      frame "Slot_4_PXIe4139" {
        n36 = Build Array("Channel Name 0") -> (w398:string[])
        n37 = Build Array("Activate Channel 0") -> (w399:bool[])
        n38 = Build Array("voltage level channel 0") -> (w400:dbl[])
        n39 = Build Array("Current Reset Value 0") -> (w389:dbl[])
        n40 = case shown="True" "Queue Power Settings" {
          tunnel: w393 -> [w408 w422]
          tunnel: refnum<k15> "Slot_4_PXIe4139" ("resource name") -> [_ w411]
          tunnel: w399 -> [_ w437]
          tunnel: w398 -> [_ w435]
          tunnel: w401 -> [w407 w410]
          tunnel: [w407 w420] -> w395
          tunnel: [w408 w419] -> w396
          tunnel: w400 -> [_ w436]
          tunnel: [w406 FALSE] -> w392
          tunnel: w391 -> [w406 _]
          tunnel: w389 -> [_ w409]
          frame False {
          }
          frame True {
            # "This is the main block here: Takes the channels that are active, their voltages, and user defined name to determine the active channels on the instrument which is compared to the initial instrument array that is passed through it. The device capture time, current limit, record length are also configured here. This outputs the parameters of all channels, their voltages, names, if active, their current limit, and the time between records. This data will be put into a cluster which is then put into an array of DCPower Instruments. This array of instruments will be used to sample DUTs especially for latchup testing. These parameters will be recorded in a output config csv in a later part of the overall project."
            # "Checking if there are any active channels in this instrument"
            # "Could I have put all of this into a subVI? Yes. I didn't though because I didn't have an elegant way to make this into a type def based on each instrument having a different number of channels. Can go into the instrument config and make another subVI that creates another parameter of interest"
            # "Can't make a type def for this unless I do something elaborate for the toggling of channels active which I don't think I can do because each instrument has a different  number of channels which doesn't lend itself to making a type def"
            # "Test if this works properly"
            n41 = call "DCPower_ConfigureInstrument.vi"("IVI Refnum in"=w411, "current limit"="current limit (A) 3", "Aperture Time"="Aperture Time (s)", "Measure Record Length"="Measure Record Length", "Active Channels Input"=w437, "Channel Name Array"=w435, "error in (no error)"=w410, "Voltage Array Input"=w436, "DCPowerInformationClusterArray_Input"=w422) -> ("Active Channels Indicator"=→"Active Channels Indicator 3":bool[], "All Channel Numbers Array"=w413:string[], "Total Voltage Indicator Array"=→"Voltage Array":dbl[], "Active Channel Numbers String List"=w414:string, "IVI Ref index"=w418:i32, "IVI Refnum out"=w430:refnum<k15>, "Active Channel Numbers Array"=w416:string[], "Active Channel Names Array"=w428:string[], "Active Channel Current Limit Array"=w427:dbl[], "Active Channel Measure Record Delta Time Array"=w426:dbl[], "Active Channel Voltage Array"=w429:dbl[], "IVI Ref Present?"=w417:bool, "error out"=w421:errorcluster)  [unwired: 4 in, 2 out]
            "All Channel Numbers Array 3" <- w413
            "Active Channel Numbers Array 3" <- w416
            "Active Channel Names Array" <- w428
            "Active Channel Voltage Array 3" <- w429
            n42 = Bundle("IVI Refnum out"=w430, "Active Channel Numbers String List"=w414, "Active Channel Numbers Array"=w416, "Active Channel Voltage Array"=w429, "Active Channel Names Array"=w428, "Active Channel Current Limit Array"=w427, "Active Channel Measure Record Delta Time Array"=w426, "All Channel Numbers Array"=w413, w409) -> (w423:T12)  [unwired: 1 in]
            n43 = Equal?(x=w414, y="") -> (x = y?=w424:bool)
            n44 = disable-structure shown="Enabled" {
              disable-tunnel: w424 -> [w445 w480]
              disable-tunnel: w423 -> [w444 w483]
              disable-tunnel: w422 -> [w443 w484]
              disable-tunnel: w421 -> [w442 w479]
              disable-tunnel: [w441 w477] -> w420
              disable-tunnel: [w440 w478] -> w419
              disable-tunnel: w418 -> [w439 w482]
              disable-tunnel: w417 -> [w438 w481]
              frame Disabled {
                # "Adding or removing from the array if there are active channels or not"
                n45 = case shown="False" w445 {
                  tunnel: w438 -> [w452 w469]
                  tunnel: [w451 w466] -> w440
                  tunnel: [w450 w467] -> w441
                  tunnel: w442 -> [w449 w464]
                  tunnel: w439 -> [w448 w468]
                  tunnel: w444 -> [w447 w462]
                  tunnel: w443 -> [w446 w470]
                  frame False {
                    # "There are active channels"
                    n46 = case shown="True" w452 {
                      tunnel: w446 -> [w455 w461]
                      tunnel: w447 -> [w454 w460]
                      tunnel: w448 -> [_ w459]
                      tunnel: w449 -> [w456 w458]
                      tunnel: [w456 w458] -> w450
                      tunnel: [w453 w457] -> w451
                      frame False {
                        # "Instantiating the instrument into the array of instruments"
                        n47 = Insert Into Array(array=w455, new element=w454) -> (w453:T1[])  [unwired: 1 in]
                      }
                      frame True {
                        # "Updating the instrument with the new configuration"
                        n48 = Replace Array Subset(array=w461, new element=w460, index=w459) -> (w457:T1[])
                      }
                    }
                  }
                  frame True {
                    # "No active channels on the instrument currently"
                    n49 = Unbundle(w462) -> ("IVI Refnum out"=w465:refnum<k15>)  [unwired: 8 out]
                    n50 = call <instrlib>:"niDCPower Close.vi"("error in (no error)"=w464, "instrument handle"=w465) -> ("error out"=w463:errorcluster)  [unwired: 9 in]
                    n51 = case shown="False" w469 {
                      tunnel: w470 -> [w472 w476]
                      tunnel: w468 -> [_ w475]
                      tunnel: [w471 w474] -> w467
                      tunnel: w463 -> [w471 w474]
                      tunnel: [w472 w473] -> w466
                      frame False {
                        # "The instrument wasn't active and it is still not being used"
                      }
                      frame True {
                        # "The instrument was active but now it is not being used"
                        n52 = Delete From Array(array=w476, index=w475) -> (array with subset deleted=w473:T1[])  [unwired: 1 in, 1 out]
                      }
                    }
                  }
                }
              }
              frame Enabled {
                n53 = disable-structure shown="Enabled" {
                  disable-tunnel: w480 -> [w492 _ _]
                  disable-tunnel: w483 -> [w491 w530 w541]
                  disable-tunnel: w484 -> [w490 w529 w544]
                  disable-tunnel: w479 -> [w489 w528 w542]
                  disable-tunnel: [w488 w527 w543] -> w477
                  disable-tunnel: [w487 w526 _] -> w478
                  disable-tunnel: w482 -> [w486 w525 _]
                  disable-tunnel: w481 -> [w485 w524 _]
                  frame Disabled {
                    # "Original (v3) version where the array had only active channels"
                    # "Adding or removing from the array if there are active channels or not"
                    n54 = case shown="False" w492 {
                      tunnel: w485 -> [w499 w516]
                      tunnel: [w498 w513] -> w487
                      tunnel: [w497 w514] -> w488
                      tunnel: w489 -> [w496 w511]
                      tunnel: w486 -> [w495 w515]
                      tunnel: w491 -> [w494 w509]
                      tunnel: w490 -> [w493 w517]
                      frame False {
                        # "There are active channels"
                        n55 = case shown="False" w499 {
                          tunnel: w493 -> [w502 w508]
                          tunnel: w494 -> [w501 w507]
                          tunnel: w495 -> [_ w506]
                          tunnel: w496 -> [w503 w505]
                          tunnel: [w503 w505] -> w497
                          tunnel: [w500 w504] -> w498
                          frame False {
                            # "Instantiating the instrument into the array of instruments"
                            n56 = Insert Into Array(array=w502, new element=w501) -> (w500:T1[])  [unwired: 1 in]
                          }
                          frame True {
                            # "Updating the instrument with the new configuration"
                            n57 = Replace Array Subset(array=w508, new element=w507, index=w506) -> (w504:T1[])
                          }
                        }
                      }
                      frame True {
                        # "No active channels on the instrument currently"
                        n58 = Unbundle(w509) -> ("IVI Refnum out"=w512:refnum<k15>)  [unwired: 8 out]
                        n59 = call <instrlib>:"niDCPower Close.vi"("error in (no error)"=w511, "instrument handle"=w512) -> ("error out"=w510:errorcluster)  [unwired: 9 in]
                        n60 = case shown="True" w516 {
                          tunnel: w517 -> [w519 w523]
                          tunnel: w515 -> [_ w522]
                          tunnel: [w518 w521] -> w514
                          tunnel: w510 -> [w518 w521]
                          tunnel: [w519 w520] -> w513
                          frame False {
                            # "The instrument wasn't active and it is still not being used"
                          }
                          frame True {
                            # "The instrument was active but now it is not being used"
                            n61 = Delete From Array(array=w523, index=w522) -> (array with subset deleted=w520:T1[])  [unwired: 1 in, 1 out]
                          }
                        }
                      }
                    }
                  }
                  frame Enabled {
                    # "v4. not removing instances with non active channels in this stage this will be in the update block outside"
                    # "Updating or instantiating the DCPower array with channel information"
                    n62 = case shown="False" w524 {
                      tunnel: w529 -> [w533 w539]
                      tunnel: w530 -> [w532 w538]
                      tunnel: w525 -> [_ w537]
                      tunnel: w528 -> [w534 w536]
                      tunnel: [w534 w536] -> w527
                      tunnel: [w531 w535] -> w526
                      frame False {
                        # "Instantiating the instrument into the array of instruments"
                        n63 = Insert Into Array(array=w533, new element=w532) -> (w531:T1[])  [unwired: 1 in]
                      }
                      frame True {
                        # "Updating the instrument with the new configuration"
                        n64 = Replace Array Subset(array=w539, new element=w538, index=w537) -> (w535:T1[])
                      }
                    }
                  }
                  frame Disabled {
                    n65 = for {
                      tunnel: w544 -> [w550] mode=indexing
                      shift-right: [w549] -> w543
                      shift-left: w542 -> [w549]
                      tunnel: w541 -> [w547]
                      tunnel: FALSE -> [w545]
                      n66 = Unbundle By Name(w547) -> ("IVI Refnum out"=w546:refnum<k15>)
                      n67 = Unbundle By Name(w550) -> ("IVI Refnum out"=w548:refnum<k15>)
                      n68 = Equal?(x=w548, y=w546) -> ()  [unwired: 1 out]
                      n69 = case shown="True" w545 {
                        frame False {
                        }
                        frame True {
                        }
                      }
                    }
                  }
                }
              }
            }
          }
        }
      }
      frame "Slot_5_PXIe4139" {
        n70 = Build Array("Channel Name 0") -> (w560:string[])
        n71 = Build Array("Activate Channel 0") -> (w561:bool[])
        n72 = Build Array("voltage level channel 0") -> (w562:dbl[])
        n73 = Build Array("Current Reset Value 0") -> (w551:dbl[])
        n74 = case shown="True" "Queue Power Settings" {
          tunnel: w555 -> [w570 w584]
          tunnel: refnum<k15> "Slot_5_PXIe4139" ("resource name") -> [_ w572]
          tunnel: w561 -> [_ w599]
          tunnel: w560 -> [_ w597]
          tunnel: w563 -> [w569 w573]
          tunnel: [w569 w582] -> w557
          tunnel: [w570 w581] -> w558
          tunnel: w562 -> [_ w598]
          tunnel: w554 -> [w568 _]
          tunnel: [w568 FALSE] -> w553
          tunnel: w551 -> [_ w571]
          frame False {
          }
          frame True {
            # "This is the main block here: Takes the channels that are active, their voltages, and user defined name to determine the active channels on the instrument which is compared to the initial instrument array that is passed through it. The device capture time, current limit, record length are also configured here. This outputs the parameters of all channels, their voltages, names, if active, their current limit, and the time between records. This data will be put into a cluster which is then put into an array of DCPower Instruments. This array of instruments will be used to sample DUTs especially for latchup testing. These parameters will be recorded in a output config csv in a later part of the overall project."
            # "Checking if there are any active channels in this instrument"
            # "Could I have put all of this into a subVI? Yes. I didn't though because I didn't have an elegant way to make this into a type def based on each instrument having a different number of channels. Can go into the instrument config and make another subVI that creates another parameter of interest"
            # "Can't make a type def for this unless I do something elaborate for the toggling of channels active which I don't think I can do because each instrument has a different  number of channels which doesn't lend itself to making a type def"
            # "Test if this works properly"
            n75 = call "DCPower_ConfigureInstrument.vi"("IVI Refnum in"=w572, "current limit"="current limit (A) 4", "Aperture Time"="Aperture Time (s)", "Measure Record Length"="Measure Record Length", "Active Channels Input"=w599, "Channel Name Array"=w597, "error in (no error)"=w573, "Voltage Array Input"=w598, "DCPowerInformationClusterArray_Input"=w584) -> ("Active Channels Indicator"=→"Active Channels Indicator 4":bool[], "All Channel Numbers Array"=w575:string[], "Total Voltage Indicator Array"=→"Voltage Array":dbl[], "Active Channel Numbers String List"=w576:string, "IVI Ref index"=w580:i32, "IVI Refnum out"=w592:refnum<k15>, "Active Channel Numbers Array"=w578:string[], "Active Channel Names Array"=w590:string[], "Active Channel Current Limit Array"=w589:dbl[], "Active Channel Measure Record Delta Time Array"=w588:dbl[], "Active Channel Voltage Array"=w591:dbl[], "IVI Ref Present?"=w579:bool, "error out"=w583:errorcluster)  [unwired: 4 in, 2 out]
            "All Channel Numbers Array 4" <- w575
            "Active Channel Numbers Array 4" <- w578
            "Active Channel Names Array" <- w590
            "Active Channel Voltage Array 4" <- w591
            n76 = Bundle("IVI Refnum out"=w592, "Active Channel Numbers String List"=w576, "Active Channel Numbers Array"=w578, "Active Channel Voltage Array"=w591, "Active Channel Names Array"=w590, "Active Channel Current Limit Array"=w589, "Active Channel Measure Record Delta Time Array"=w588, "All Channel Numbers Array"=w575, w571) -> (w585:T12)  [unwired: 1 in]
            n77 = Equal?(x=w576, y="") -> (x = y?=w586:bool)
            n78 = disable-structure shown="Enabled" {
              disable-tunnel: w586 -> [w607 w641]
              disable-tunnel: w585 -> [w606 w645]
              disable-tunnel: w584 -> [w605 w646]
              disable-tunnel: w583 -> [w604 w642]
              disable-tunnel: [w603 w640] -> w582
              disable-tunnel: [w602 w639] -> w581
              disable-tunnel: w580 -> [w601 w644]
              disable-tunnel: w579 -> [w600 w643]
              frame Disabled {
                # "Adding or removing from the array if there are active channels or not"
                n79 = case shown="False" w607 {
                  tunnel: w600 -> [w614 w631]
                  tunnel: [w613 w628] -> w602
                  tunnel: [w612 w629] -> w603
                  tunnel: w604 -> [w611 w626]
                  tunnel: w601 -> [w610 w630]
                  tunnel: w606 -> [w609 w624]
                  tunnel: w605 -> [w608 w632]
                  frame False {
                    # "There are active channels"
                    n80 = case shown="True" w614 {
                      tunnel: w608 -> [w617 w623]
                      tunnel: w609 -> [w616 w622]
                      tunnel: w610 -> [_ w621]
                      tunnel: w611 -> [w618 w620]
                      tunnel: [w618 w620] -> w612
                      tunnel: [w615 w619] -> w613
                      frame False {
                        # "Instantiating the instrument into the array of instruments"
                        n81 = Insert Into Array(array=w617, new element=w616) -> (w615:T1[])  [unwired: 1 in]
                      }
                      frame True {
                        # "Updating the instrument with the new configuration"
                        n82 = Replace Array Subset(array=w623, new element=w622, index=w621) -> (w619:T1[])
                      }
                    }
                  }
                  frame True {
                    # "No active channels on the instrument currently"
                    n83 = Unbundle(w624) -> ("IVI Refnum out"=w627:refnum<k15>)  [unwired: 8 out]
                    n84 = call <instrlib>:"niDCPower Close.vi"("error in (no error)"=w626, "instrument handle"=w627) -> ("error out"=w625:errorcluster)  [unwired: 9 in]
                    n85 = case shown="False" w631 {
                      tunnel: w632 -> [w634 w638]
                      tunnel: w630 -> [_ w637]
                      tunnel: [w633 w636] -> w629
                      tunnel: w625 -> [w633 w636]
                      tunnel: [w634 w635] -> w628
                      frame False {
                        # "The instrument wasn't active and it is still not being used"
                      }
                      frame True {
                        # "The instrument was active but now it is not being used"
                        n86 = Delete From Array(array=w638, index=w637) -> (array with subset deleted=w635:T1[])  [unwired: 1 in, 1 out]
                      }
                    }
                  }
                }
              }
              frame Enabled {
                n87 = disable-structure shown="Enabled" {
                  disable-tunnel: w641 -> [w654 _ _]
                  disable-tunnel: w645 -> [w653 w692 w703]
                  disable-tunnel: w646 -> [w652 w691 w706]
                  disable-tunnel: w642 -> [w651 w690 w704]
                  disable-tunnel: [w650 w689 w705] -> w640
                  disable-tunnel: [w649 w688 _] -> w639
                  disable-tunnel: w644 -> [w648 w687 _]
                  disable-tunnel: w643 -> [w647 w686 _]
                  frame Disabled {
                    # "Original (v3) version where the array had only active channels"
                    # "Adding or removing from the array if there are active channels or not"
                    n88 = case shown="False" w654 {
                      tunnel: w647 -> [w661 w678]
                      tunnel: [w660 w675] -> w649
                      tunnel: [w659 w676] -> w650
                      tunnel: w651 -> [w658 w673]
                      tunnel: w648 -> [w657 w677]
                      tunnel: w653 -> [w656 w671]
                      tunnel: w652 -> [w655 w679]
                      frame False {
                        # "There are active channels"
                        n89 = case shown="False" w661 {
                          tunnel: w655 -> [w664 w670]
                          tunnel: w656 -> [w663 w669]
                          tunnel: w657 -> [_ w668]
                          tunnel: w658 -> [w665 w667]
                          tunnel: [w665 w667] -> w659
                          tunnel: [w662 w666] -> w660
                          frame False {
                            # "Instantiating the instrument into the array of instruments"
                            n90 = Insert Into Array(array=w664, new element=w663) -> (w662:T1[])  [unwired: 1 in]
                          }
                          frame True {
                            # "Updating the instrument with the new configuration"
                            n91 = Replace Array Subset(array=w670, new element=w669, index=w668) -> (w666:T1[])
                          }
                        }
                      }
                      frame True {
                        # "No active channels on the instrument currently"
                        n92 = Unbundle(w671) -> ("IVI Refnum out"=w674:refnum<k15>)  [unwired: 8 out]
                        n93 = call <instrlib>:"niDCPower Close.vi"("error in (no error)"=w673, "instrument handle"=w674) -> ("error out"=w672:errorcluster)  [unwired: 9 in]
                        n94 = case shown="True" w678 {
                          tunnel: w679 -> [w681 w685]
                          tunnel: w677 -> [_ w684]
                          tunnel: [w680 w683] -> w676
                          tunnel: w672 -> [w680 w683]
                          tunnel: [w681 w682] -> w675
                          frame False {
                            # "The instrument wasn't active and it is still not being used"
                          }
                          frame True {
                            # "The instrument was active but now it is not being used"
                            n95 = Delete From Array(array=w685, index=w684) -> (array with subset deleted=w682:T1[])  [unwired: 1 in, 1 out]
                          }
                        }
                      }
                    }
                  }
                  frame Enabled {
                    # "v4. not removing instances with non active channels in this stage this will be in the update block outside"
                    # "Updating or instantiating the DCPower array with channel information"
                    n96 = case shown="True" w686 {
                      tunnel: w691 -> [w695 w701]
                      tunnel: w692 -> [w694 w700]
                      tunnel: w687 -> [_ w699]
                      tunnel: w690 -> [w696 w698]
                      tunnel: [w696 w698] -> w689
                      tunnel: [w693 w697] -> w688
                      frame False {
                        # "Instantiating the instrument into the array of instruments"
                        n97 = Insert Into Array(array=w695, new element=w694) -> (w693:T1[])  [unwired: 1 in]
                      }
                      frame True {
                        # "Updating the instrument with the new configuration"
                        n98 = Replace Array Subset(array=w701, new element=w700, index=w699) -> (w697:T1[])
                      }
                    }
                  }
                  frame Disabled {
                    n99 = for {
                      tunnel: w706 -> [w712] mode=indexing
                      shift-right: [w711] -> w705
                      shift-left: w704 -> [w711]
                      tunnel: w703 -> [w709]
                      tunnel: FALSE -> [w707]
                      n100 = Unbundle By Name(w709) -> ("IVI Refnum out"=w708:refnum<k15>)
                      n101 = Unbundle By Name(w712) -> ("IVI Refnum out"=w710:refnum<k15>)
                      n102 = Equal?(x=w710, y=w708) -> ()  [unwired: 1 out]
                      n103 = case shown="True" w707 {
                        frame False {
                        }
                        frame True {
                        }
                      }
                    }
                  }
                }
              }
            }
          }
        }
      }
      frame "Slot_6_PXIe4139" {
        n104 = Build Array("Channel Name 0") -> (w722:string[])
        n105 = Build Array("Activate Channel 0") -> (w723:bool[])
        n106 = Build Array("voltage level channel 0") -> (w724:dbl[])
        n107 = Build Array("Current Reset Value 0") -> (w713:dbl[])
        n108 = case shown="True" "Queue Power Settings" {
          tunnel: w717 -> [w732 w746]
          tunnel: refnum<k15> "Slot_6_PXIe4139" ("resource name") -> [_ w735]
          tunnel: w723 -> [_ w761]
          tunnel: w722 -> [_ w759]
          tunnel: w725 -> [w731 w734]
          tunnel: [w731 w744] -> w719
          tunnel: [w732 w743] -> w720
          tunnel: w724 -> [_ w760]
          tunnel: [w730 FALSE] -> w716
          tunnel: w715 -> [w730 _]
          tunnel: w713 -> [_ w733]
          frame False {
          }
          frame True {
            # "This is the main block here: Takes the channels that are active, their voltages, and user defined name to determine the active channels on the instrument which is compared to the initial instrument array that is passed through it. The device capture time, current limit, record length are also configured here. This outputs the parameters of all channels, their voltages, names, if active, their current limit, and the time between records. This data will be put into a cluster which is then put into an array of DCPower Instruments. This array of instruments will be used to sample DUTs especially for latchup testing. These parameters will be recorded in a output config csv in a later part of the overall project."
            # "Checking if there are any active channels in this instrument"
            # "Could I have put all of this into a subVI? Yes. I didn't though because I didn't have an elegant way to make this into a type def based on each instrument having a different number of channels. Can go into the instrument config and make another subVI that creates another parameter of interest"
            # "Can't make a type def for this unless I do something elaborate for the toggling of channels active which I don't think I can do because each instrument has a different  number of channels which doesn't lend itself to making a type def"
            # "Test if this works properly"
            n109 = call "DCPower_ConfigureInstrument.vi"("IVI Refnum in"=w735, "current limit"="current limit (A)", "Aperture Time"="Aperture Time (s)", "Measure Record Length"="Measure Record Length", "Active Channels Input"=w761, "Channel Name Array"=w759, "error in (no error)"=w734, "Voltage Array Input"=w760, "DCPowerInformationClusterArray_Input"=w746) -> ("Active Channels Indicator"=→"Active Channels Indicator":bool[], "All Channel Numbers Array"=w737:string[], "Total Voltage Indicator Array"=→"Voltage Array":dbl[], "Active Channel Numbers String List"=w738:string, "IVI Ref index"=w742:i32, "IVI Refnum out"=w754:refnum<k15>, "Active Channel Numbers Array"=w740:string[], "Active Channel Names Array"=w752:string[], "Active Channel Current Limit Array"=w751:dbl[], "Active Channel Measure Record Delta Time Array"=w750:dbl[], "Active Channel Voltage Array"=w753:dbl[], "IVI Ref Present?"=w741:bool, "error out"=w745:errorcluster)  [unwired: 4 in, 2 out]
            "All Channel Numbers Array" <- w737
            "Active Channel Numbers Array" <- w740
            "Active Channel Names Array" <- w752
            "Active Channel Voltage Array" <- w753
            n110 = Bundle("IVI Refnum out"=w754, "Active Channel Numbers String List"=w738, "Active Channel Numbers Array"=w740, "Active Channel Voltage Array"=w753, "Active Channel Names Array"=w752, "Active Channel Current Limit Array"=w751, "Active Channel Measure Record Delta Time Array"=w750, "All Channel Numbers Array"=w737, w733) -> (w747:T12)  [unwired: 1 in]
            n111 = Equal?(x=w738, y="") -> (x = y?=w748:bool)
            n112 = disable-structure shown="Enabled" {
              disable-tunnel: w748 -> [w769 w803]
              disable-tunnel: w747 -> [w768 w807]
              disable-tunnel: w746 -> [w767 w808]
              disable-tunnel: w745 -> [w766 w804]
              disable-tunnel: [w765 w802] -> w744
              disable-tunnel: [w764 w801] -> w743
              disable-tunnel: w742 -> [w763 w806]
              disable-tunnel: w741 -> [w762 w805]
              frame Disabled {
                # "Adding or removing from the array if there are active channels or not"
                n113 = case shown="False" w769 {
                  tunnel: w762 -> [w776 w793]
                  tunnel: [w775 w790] -> w764
                  tunnel: [w774 w791] -> w765
                  tunnel: w766 -> [w773 w788]
                  tunnel: w763 -> [w772 w792]
                  tunnel: w768 -> [w771 w786]
                  tunnel: w767 -> [w770 w794]
                  frame False {
                    # "There are active channels"
                    n114 = case shown="True" w776 {
                      tunnel: w770 -> [w779 w785]
                      tunnel: w771 -> [w778 w784]
                      tunnel: w772 -> [_ w783]
                      tunnel: w773 -> [w780 w782]
                      tunnel: [w780 w782] -> w774
                      tunnel: [w777 w781] -> w775
                      frame False {
                        # "Instantiating the instrument into the array of instruments"
                        n115 = Insert Into Array(array=w779, new element=w778) -> (w777:T1[])  [unwired: 1 in]
                      }
                      frame True {
                        # "Updating the instrument with the new configuration"
                        n116 = Replace Array Subset(array=w785, new element=w784, index=w783) -> (w781:T1[])
                      }
                    }
                  }
                  frame True {
                    # "No active channels on the instrument currently"
                    n117 = Unbundle(w786) -> ("IVI Refnum out"=w789:refnum<k15>)  [unwired: 8 out]
                    n118 = call <instrlib>:"niDCPower Close.vi"("error in (no error)"=w788, "instrument handle"=w789) -> ("error out"=w787:errorcluster)  [unwired: 9 in]
                    n119 = case shown="False" w793 {
                      tunnel: w794 -> [w796 w800]
                      tunnel: w792 -> [_ w799]
                      tunnel: [w795 w798] -> w791
                      tunnel: w787 -> [w795 w798]
                      tunnel: [w796 w797] -> w790
                      frame False {
                        # "The instrument wasn't active and it is still not being used"
                      }
                      frame True {
                        # "The instrument was active but now it is not being used"
                        n120 = Delete From Array(array=w800, index=w799) -> (array with subset deleted=w797:T1[])  [unwired: 1 in, 1 out]
                      }
                    }
                  }
                }
              }
              frame Enabled {
                n121 = disable-structure shown="Enabled" {
                  disable-tunnel: w803 -> [w816 _ _]
                  disable-tunnel: w807 -> [w815 w854 w865]
                  disable-tunnel: w808 -> [w814 w853 w868]
                  disable-tunnel: w804 -> [w813 w852 w866]
                  disable-tunnel: [w812 w851 w867] -> w802
                  disable-tunnel: [w811 w850 _] -> w801
                  disable-tunnel: w806 -> [w810 w849 _]
                  disable-tunnel: w805 -> [w809 w848 _]
                  frame Disabled {
                    # "Original (v3) version where the array had only active channels"
                    # "Adding or removing from the array if there are active channels or not"
                    n122 = case shown="False" w816 {
                      tunnel: w809 -> [w823 w840]
                      tunnel: [w822 w837] -> w811
                      tunnel: [w821 w838] -> w812
                      tunnel: w813 -> [w820 w835]
                      tunnel: w810 -> [w819 w839]
                      tunnel: w815 -> [w818 w833]
                      tunnel: w814 -> [w817 w841]
                      frame False {
                        # "There are active channels"
                        n123 = case shown="False" w823 {
                          tunnel: w817 -> [w826 w832]
                          tunnel: w818 -> [w825 w831]
                          tunnel: w819 -> [_ w830]
                          tunnel: w820 -> [w827 w829]
                          tunnel: [w827 w829] -> w821
                          tunnel: [w824 w828] -> w822
                          frame False {
                            # "Instantiating the instrument into the array of instruments"
                            n124 = Insert Into Array(array=w826, new element=w825) -> (w824:T1[])  [unwired: 1 in]
                          }
                          frame True {
                            # "Updating the instrument with the new configuration"
                            n125 = Replace Array Subset(array=w832, new element=w831, index=w830) -> (w828:T1[])
                          }
                        }
                      }
                      frame True {
                        # "No active channels on the instrument currently"
                        n126 = Unbundle(w833) -> ("IVI Refnum out"=w836:refnum<k15>)  [unwired: 8 out]
                        n127 = call <instrlib>:"niDCPower Close.vi"("error in (no error)"=w835, "instrument handle"=w836) -> ("error out"=w834:errorcluster)  [unwired: 9 in]
                        n128 = case shown="True" w840 {
                          tunnel: w841 -> [w843 w847]
                          tunnel: w839 -> [_ w846]
                          tunnel: [w842 w845] -> w838
                          tunnel: w834 -> [w842 w845]
                          tunnel: [w843 w844] -> w837
                          frame False {
                            # "The instrument wasn't active and it is still not being used"
                          }
                          frame True {
                            # "The instrument was active but now it is not being used"
                            n129 = Delete From Array(array=w847, index=w846) -> (array with subset deleted=w844:T1[])  [unwired: 1 in, 1 out]
                          }
                        }
                      }
                    }
                  }
                  frame Enabled {
                    # "v4. not removing instances with non active channels in this stage this will be in the update block outside"
                    # "Updating or instantiating the DCPower array with channel information"
                    n130 = case shown="False" w848 {
                      tunnel: w853 -> [w857 w863]
                      tunnel: w854 -> [w856 w862]
                      tunnel: w849 -> [_ w861]
                      tunnel: w852 -> [w858 w860]
                      tunnel: [w858 w860] -> w851
                      tunnel: [w855 w859] -> w850
                      frame False {
                        # "Instantiating the instrument into the array of instruments"
                        n131 = Insert Into Array(array=w857, new element=w856) -> (w855:T1[])  [unwired: 1 in]
                      }
                      frame True {
                        # "Updating the instrument with the new configuration"
                        n132 = Replace Array Subset(array=w863, new element=w862, index=w861) -> (w859:T1[])
                      }
                    }
                  }
                  frame Disabled {
                    n133 = for {
                      tunnel: w868 -> [w874] mode=indexing
                      shift-right: [w873] -> w867
                      shift-left: w866 -> [w873]
                      tunnel: w865 -> [w871]
                      tunnel: FALSE -> [w869]
                      n134 = Unbundle By Name(w871) -> ("IVI Refnum out"=w870:refnum<k15>)
                      n135 = Unbundle By Name(w874) -> ("IVI Refnum out"=w872:refnum<k15>)
                      n136 = Equal?(x=w872, y=w870) -> ()  [unwired: 1 out]
                      n137 = case shown="True" w869 {
                        frame False {
                        }
                        frame True {
                        }
                      }
                    }
                  }
                }
              }
            }
          }
        }
      }
    }
    "Supplies Updated?" <- w8
    "VISAPowerInformationClusterArray" <- w28
    n138 = Array Size(array=w11) -> (size(s)=w18:i32)
    n139 = Array Size(array=w28) -> (size(s)=w17:i32)
    n140 = Not Equal To 0?(x=w18) -> (x != 0?=w15:bool)
    n141 = Not Equal To 0?(x=w17) -> (x != 0?=w16:bool)
    n142 = Or(x=w15, y=w16) -> (x .or. y?=w13:bool)
    n143 = case shown="True" "Update Changes" {
      selector: "Update Changes" -> [_ w52]
      tunnel: [w31 w45] -> w22
      tunnel: w11 -> [w31 w54]
      tunnel: w9 -> [w32 w53]
      tunnel: [w32 w44] -> w21
      tunnel: w8 -> [w30 _]
      tunnel: [w30 w52] -> w25
      tunnel: "ColorPalette" -> [_ w33]
      frame False {
      }
      frame True {
        # "Fetching some data to confirm part is powered on properly. Indicators are shown to the right"
        # "Making all the colors and names of the chart \"none\" so empty names are called \"none\""
        # "renaming the legend and the colors of the chart"
        # "closing the instrument if it is not configured anymore"
        n144 = for {
          tunnel: [w105] -> w45 mode=indexing if=w94
          tunnel: w54 -> [w105] mode=indexing
          shift-right: [w96] -> w49
          shift-left: w53 -> [w103]
          n145 = Unbundle(w105) -> ("IVI Refnum out"=w104:refnum<k15>, "Active Channel Numbers String List"=w99:string, "Active Channel Numbers Array"=w92:string[])  [unwired: 6 out]
          n146 = Equal?(x=w99, y="") -> (x = y?=w95:bool)
          n147 = call "StringArray2StringList.vi"("String Array"=w92) -> ("String List"=w98:string)
          n148 = call <instrlib>:"niDCPower Initiate With Channels.vi"("error in (no error)"=w103, "channel name"=w98, "instrument handle"=w104) -> ("error out"=w102:errorcluster, "instrument handle out"=w101:refnum<k15>)  [unwired: 7 in]
          n149 = call <instrlib>:"niDCPower Abort With Channels.vi"("error in (no error)"=w102, "channel name"=w98, "instrument handle"=w101) -> ("error out"=w97:errorcluster, "instrument handle out"=w93:refnum<k15>)  [unwired: 7 in]
          n150 = case shown="True" w95 {
            tunnel: w97 -> [w106 w109]
            tunnel: [w106 w107] -> w96
            tunnel: w93 -> [_ w108]
            frame False {
            }
            frame True {
              n151 = call <instrlib>:"niDCPower Close.vi"("error in (no error)"=w109, "instrument handle"=w108) -> ("error out"=w107:errorcluster)  [unwired: 9 in]
            }
          }
          n152 = Not(x=w95) -> (.not. x?=w94:bool)
        }
        "DCPowerInformationClusterArray" <- w45
        n153 = for {
          tunnel: w45 -> [w91] mode=indexing
          shift-right: [w88] -> w50
          shift-left: w49 -> [w87]
          n154 = Unbundle By Name(w91) -> ("IVI Refnum out"=w89:refnum<k15>, "Active Channel Numbers String List"=w90:string)
          n155 = call <instrlib>:"niDCPower Initiate With Channels.vi"("error in (no error)"=w87, "channel name"=w90, "instrument handle"=w89) -> ("error out"=w88:errorcluster)  [unwired: 7 in, 1 out]
        }
        n156 = call "Convert_InstrumentReferenceArray_2_ChannelReferenceArray.vi"("error in (no error)"=w50, "DCPowerInformationClusterArray_Input"=w45) -> ("error out"=w47:errorcluster, "DCPowerInformationArrayOutput"=w46:T13)
        n157 = for {
          shift-right: [w81] -> w48
          shift-left: w47 -> [w79]
          tunnel: w33 -> [_] mode=indexing
          i -> [w78]
          w77 = "NONE" ("Plot.Plot Name")
          n158 = property on="Current Waveform Array" class="WFChart (strict)"(error in=w79, "Active Plot"=w78, "Plot.Plot Name"=w77) -> (error out=w80:errorcluster)  [unwired: 1 in, 1 out]
          n159 = property on="Voltage Waveform Array" class="WFChart (strict)"(error in=w80, "Active Plot"=w78, "Plot.Plot Name"=w77) -> (error out=w81:errorcluster)  [unwired: 1 in, 1 out]
        }
        n160 = case shown="No Error" w48 {
          selector: w48 -> [w75 _]
          tunnel: [w75 w76] -> w42
          tunnel: w47 -> [_ w76]
          frame No Error {
          }
          frame Error {
          }
        }
        n161 = for {
          shift-right: [w72] -> w41
          shift-left: w42 -> [w73]
          tunnel: w46 -> [w71] mode=indexing
          tunnel: w33 -> [w70] mode=indexing
          tunnel: w33 -> [w69] mode=indexing
          i -> [w68]
          n162 = Unbundle By Name(w71) -> ("Channel Name 23"=w67:string)
          n163 = property on="Current Waveform Array" class="WFChart (strict)"(error in=w73, "Active Plot"=w68, "Plot.Plot Name"=w67, "Plot.Plot Color"=w70) -> (error out=w74:errorcluster)  [unwired: 1 in, 1 out]
          n164 = property on="Voltage Waveform Array" class="WFChart (strict)"(error in=w74, "Active Plot"=w68, "Plot.Plot Name"=w67, "Plot.Plot Color"=w69) -> (error out=w72:errorcluster)  [unwired: 1 in, 1 out]
        }
        n165 = case shown="Error .." w41 {
          selector: w41 -> [w60 _]
          tunnel: [w60 w61] -> w43
          tunnel: w42 -> [_ w61]
          frame No Error {
          }
          frame Error {
          }
        }
        n166 = for {
          N: 1000 -> [_]
          tunnel: w46 -> [_]
          tunnel: timestamp(0 s since 1904-01-01) ("Initial Time") -> [w86]
          shift-right: [w84] -> w38
          shift-left: w43 -> [w85]
          tunnel: [w83] -> w40
          tunnel: [w82] -> w37
          n167 = call "Fetch&Process_Measurements_V4.vi"("Initial Time"=w86, "error in (no error)"=w85) -> ("Current Waveform Array"=w82:waveform(dbl)[], "Voltage Waveform Array"=w83:waveform(dbl)[], "error out"=w84:errorcluster)  [unwired: 6 in, 5 out]
          "Current Waveform Array" <- w82
          "Voltage Waveform Array" <- w83
        }
        n168 = for {
          tunnel: w40 -> [w59] mode=indexing
          shift-right: [w58] -> w39
          shift-left: w38 -> [w58]
          tunnel: w37 -> [w57] mode=indexing
          tunnel: [w56] -> w36 mode=indexing
          tunnel: [w55] -> w35 mode=indexing
          n169 = Unbundle By Name(w57) -> ("Y"=w55:dbl[])
          n170 = Unbundle By Name(w59) -> ("Y"=w56:dbl[])
        }
        "Voltage Measurement (V)" <- w36
        "Current Measurement (A)" <- w35
        n171 = for {
          tunnel: w45 -> [w66] mode=indexing
          shift-right: [w62] -> w44
          shift-left: w39 -> [w63]
          n172 = Unbundle By Name(w66) -> ("IVI Refnum out"=w65:refnum<k15>, "Active Channel Numbers String List"=w64:string)
          n173 = call <instrlib>:"niDCPower Abort With Channels.vi"("error in (no error)"=w63, "channel name"=w64, "instrument handle"=w65) -> ("error out"=w62:errorcluster)  [unwired: 7 in, 1 out]
        }
      }
    }
    n174 = case shown="True" "Exit SubVI" {
      selector: "Exit SubVI" -> [w110 w114]
      tunnel: w13 -> [_ w112]
      tunnel: [w110 w115] -> w12
      tunnel: w25 -> [_ w111]
      frame False {
      }
      frame True {
        n175 = And(x=w111, y=w112) -> (x .and. y?=w113:bool)
        n176 = case shown="False" w113 {
          tunnel: [w117 w120] -> w115
          tunnel: w114 -> [_ w120]
          frame False {
            n177 = Two Button Dialog(message="You need to have at least one channel configured and updated", 1:"Ok, I will stay in this VI" ("F button name (\"Cancel\")"), 2:"I don't care" ("T button name (\"OK\")")) -> (T button?=w117:bool)
          }
          frame True {
          }
        }
      }
    }
    n178 = Or(x=w21, y=w12) -> (x .or. y?=w27:bool)
  }
  "error out" <- w6
  "VISAPowerInfoOutputArray" <- w2
  "DCPowerInformationClusterArray_Output" <- w5
  n179 = disable-structure shown="Disabled" {
    disable-tunnel: _ -> [w876 _]
    disable-tunnel: _ -> [w875 _]
    frame Disabled {
      n180 = for {
        shift-right: [w877] -> _
        shift-left: w876 -> [w880]
        tunnel: w875 -> [w879] mode=indexing
        n181 = Unbundle(w879) -> ("instrument handle out"=w878)  [unwired: 4 out]
        n182 = call <instrlib>:"niDCPower Close.vi"("error in (no error)"=w880, "instrument handle"=w878) -> ("error out"=w877:errorcluster)  [unwired: 9 in]
      }
    }
    frame Enabled {
    }
  }
